vi "initializeStyleCollection.vi"(8 "error in (no error)":errorcluster, 11 "MS-Word in":refnum<class "MS-Word.lvclass">) -> (0 "error out":errorcluster, 3 "MS-Word out":refnum<class "MS-Word.lvclass">)   [LabVIEW 2017, in "LabVIEW NPOI.lvlib" / "MS-Word.lvclass"]
uses:
  MS-Word.lvclass
  Document/Document.lvclass
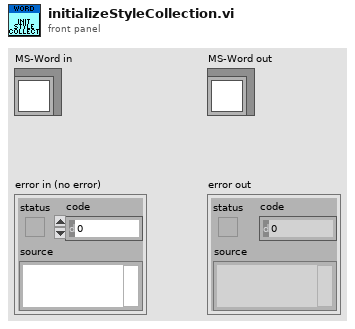
[diagram p1: front panel]
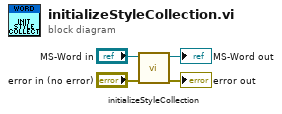
[diagram p0: block diagram]
diagram:
  n1 = call-parent "initializeStyleCollection.vi"("error in (no error)"="error in (no error)", "Document in"="MS-Word in") -> ("error out"=→"error out":errorcluster, "Document out"=→"MS-Word out":refnum<class "MS-Word.lvclass">)  [unwired: 8 in]
